vi "Resideo Set Temp.vi"(8 "error in (no error)":errorcluster, 10 "Vesta Data":T1 {"Water Heater Temp (°F)" min=32 max=203}, 11 "Modbus Master in":refnum<class "Modbus Master.lvclass">) -> (0 "error out":errorcluster, 3 "Modbus Master out":refnum<class "Modbus Master.lvclass">)   [LabVIEW 2023]
uses:
  <vilib>/NI/Modbus Library/API/Master/Modbus Master.lvclass
  Type Definitions/Temperature Control.ctl
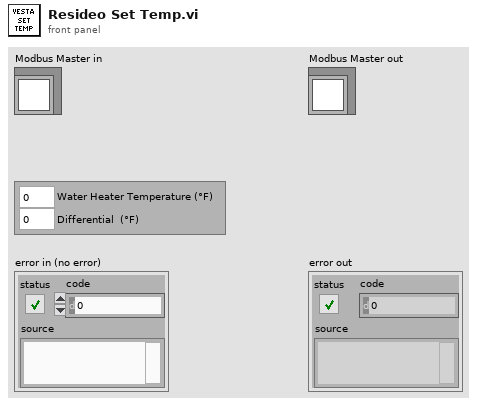
[diagram p1: front panel]
types:
  T1 = typedef "Temperature Control.ctl" = cluster{"Water Heater Temp (°F)":u16, "Differential  (°F)":dbl}
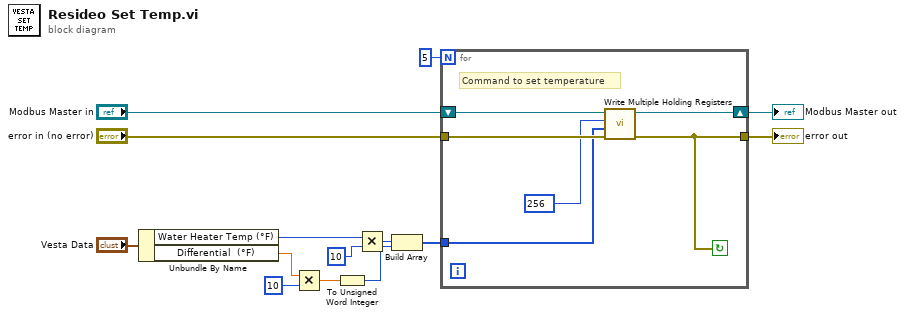
[diagram p0: block diagram]
diagram:
  n1 = Unbundle By Name("Vesta Data") -> ("Water Heater Temp (°F)"=w6:u16, "Differential  (°F)"=w4:dbl)
  n2 = Multiply(x=w4, y=u16 10) -> (x*y=w3:dbl)
  n3 = To Unsigned Word Integer(number=w3) -> (unsigned 16bit integer=w2:u16)
  n4 = Multiply(x=w6, y=u16 10) -> (x*y=w13:u16)
  n5 = Build Array(w13, w2) -> (w14:u16[])
  n6 = for {
    N: 5 -> [_]
    shift-right: [w18] -> w11
    shift-left: "Modbus Master in" -> [w19]
    tunnel: "error in (no error)" -> [w20]
    tunnel: [w16] -> w9
    tunnel: w14 -> [w15]
    stop <- w16 continue-if-true
    # "Command to set temperature"
    n7 = call-dynamic "Write Multiple Holding Registers.vi"("error in"=w20, "registers to write"=w15, "starting address"=u16 256, "Modbus master in"=w19) -> ("error out"=w16:errorcluster, "Modbus master out"=w18:refnum<class "Modbus Master.lvclass">)  [unwired: 6 in]
  }
  "Modbus Master out" <- w11
  "error out" <- w9
